vi "Player Info.vi"(8 "Victory Speech":string="Victory Comes to the Patient", 9 "Name":string="Hesitant Wolf", 11 "Hesitant Wolf in":refnum<class "Hesitant Wolf.lvclass">) -> (3 "Hesitant Wolf out":refnum<class "Hesitant Wolf.lvclass">)   [LabVIEW 2015, in "Hesitant Wolf.lvclass"]
uses:
  Hesitant Wolf.lvclass
  Square/Square.lvclass
panel:
  # "Set default values for these two string controls"
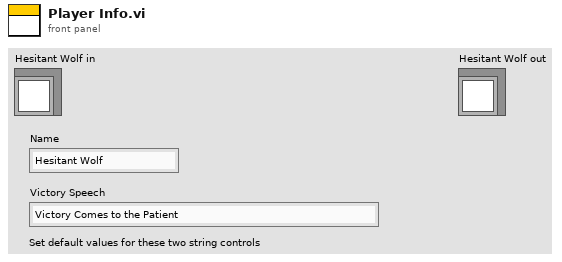
[diagram p1: front panel]
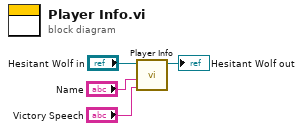
[diagram p0: block diagram]
diagram:
  n1 = call-parent "Player Info.vi"("Victory Speech"="Victory Speech", "Name"="Name", "Square in"="Hesitant Wolf in") -> ("Square out"=→"Hesitant Wolf out":refnum<class "Hesitant Wolf.lvclass">)  [unwired: 8 in]
